vi "Transfer Group.Errors.vi"   [LabVIEW 2017, in "DSF Core.lvlib" / "Transfer Group.lvclass"]
uses:
  Transfer Group.lvclass
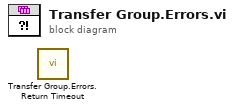
[diagram p0: block diagram]
diagram:
  n1 = call "Transfer Group.Errors.Return Timeout.vi"() -> ()  [unwired: 10 in, 2 out]
